vi "Divide Images.vi"(0 "image in":refnum<class "MSC Image.lvclass">, 1 "image 2 in":refnum<class "MSC Image.lvclass">, 2 "Scalar":dbl=1.0, 5 "error in (no error)":errorcluster) -> (14 "image out":refnum<class "MSC Image.lvclass">, 15 "image 2 out":refnum<class "MSC Image.lvclass">, 19 "error out":errorcluster)   [LabVIEW 2016, in "MSC Image.lvclass"]
doc: "image = image / image 2 / Scalar"
uses:
  MSC Image.lvclass
  Dependencies/x86/MSC I Process32.dll
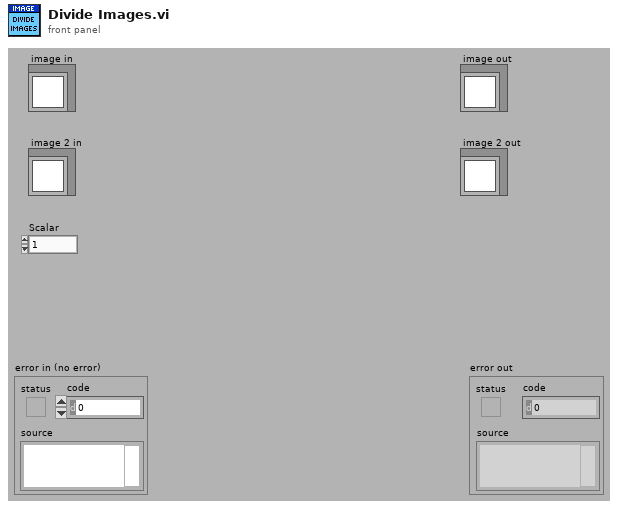
[diagram p1: front panel]
types:
  T1 = typedef "Image.ctl" = cluster{"Pointer":u64, "Size":T2, "Image Type":T3, "Time Stamp":timestamp, "Variant":variant}
  T2 = typedef "Size.ctl" = cluster{"Cols":i32, "Rows":i32}
  T3 = typedef "Image Type.ctl" = i32
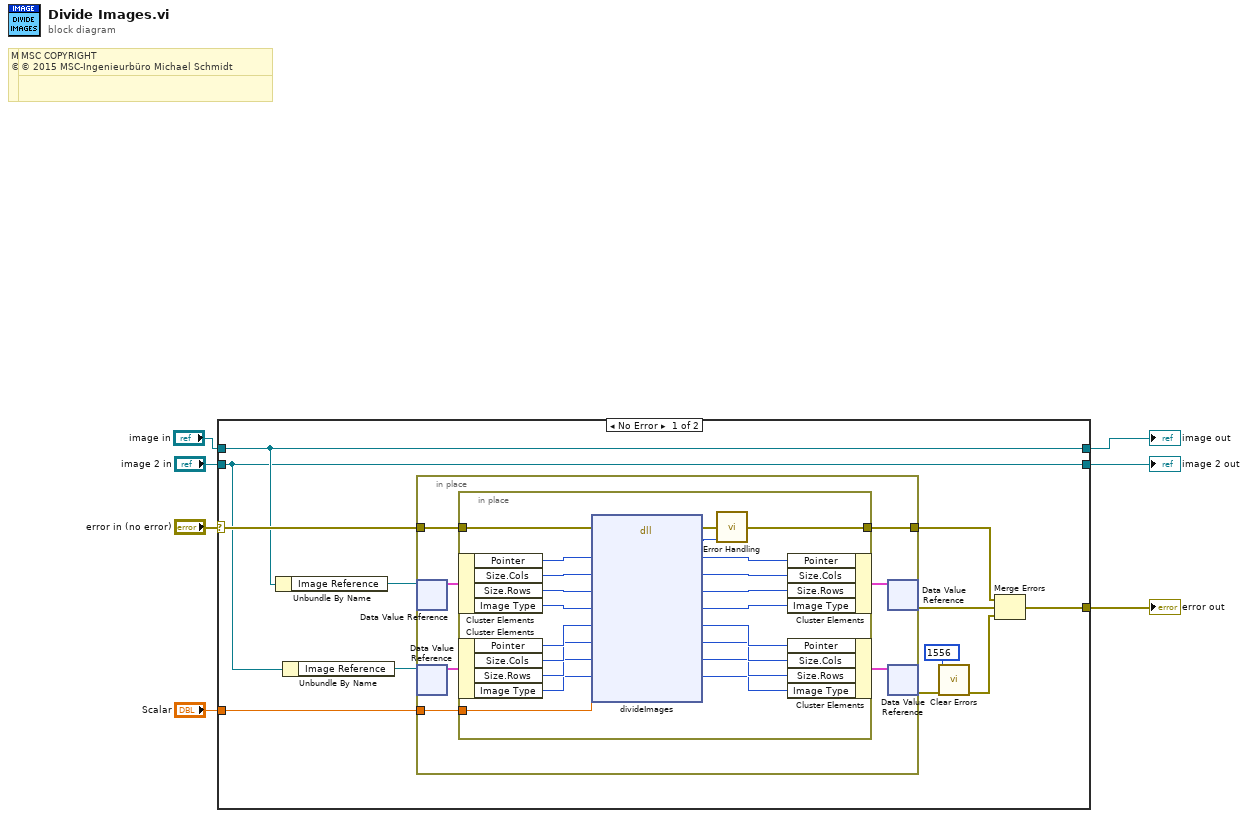
[diagram p0: block diagram]
diagram:
  # "MSC COPYRIGHT\n© 2016 MSC-Ingenieurbüro Michael Schmidt"
  # "MSC COPYRIGHT\n© 2016 MSC-Ingenieurbüro Michael Schmidt"
  # "MSC COPYRIGHT\n© 2015 MSC-Ingenieurbüro Michael Schmidt"
  # "MSC COPYRIGHT\n© 2015 MSC-Ingenieurbüro Michael Schmidt"
  n1 = case shown="No Error" "error in (no error)" {
    selector: "error in (no error)" -> [w16 w50]
    tunnel: [w19 w50] -> w3
    tunnel: [w12 w49] -> w6
    tunnel: "image in" -> [w15 w48]
    tunnel: "image 2 in" -> [w12 w49]
    tunnel: [w15 w48] -> w7
    tunnel: "Scalar" -> [w11 _]
    frame No Error {
      n2 = Unbundle By Name(w15) -> ("Image Reference"=w14:refnum<data-value>)
      n3 = Unbundle By Name(w12) -> ("Image Reference"=w13:refnum<data-value>)
      n4 = in-place {
        in-place-border: w16 -> [w24]
        in-place-border: [w23] -> w18
        in-place-border: w11 -> [w20]
        n5 = in-place-dvr #1(w14) -> (w25:T1)  [unwired: 1 out]
        n6 = in-place-dvr #2(w13) -> (w22:T1)  [unwired: 1 out]
        n7 = in-place {
          in-place-border: w24 -> [w28]
          in-place-border: [w47] -> w23
          in-place-border: w20 -> [w27]
          n8 = in-place-cluster #3(w25) -> ("Pointer"=w46:u64, "Size.Cols"=w45:i32, "Size.Rows"=w44:i32, "Image Type"=w43:T3)
          n9 = in-place-cluster #4(w22) -> ("Pointer"=w42:u64, "Size.Cols"=w41:i32, "Size.Rows"=w40:i32, "Image Type"=w39:T3)
          n10 = dll-call lib="C:/Users/MSC/LabVIEW Projekte/LV 2014/MSC I-Process/user.lib/MSC-I Process/Dependencies/x86/MSC I Process*.dll" fn="divideImages"(error in=w28, "pointer"=w46, "cols"=w45, "rows"=w44, "type"=w43, "pointer2"=w42, "cols2"=w41, "rows2"=w40, "type2"=w39, "scalar"=w27) -> (error out=w29:errorcluster, "error"=w30:i32, "pointer"=w34:u64, "cols"=w33:i32, "rows"=w32:i32, "type"=w31:i32, "pointer2"=w38:u64, "cols2"=w37:i32, "rows2"=w36:i32, "type2"=w35:i32)  [unwired: 3 in, 1 out]
          n11 = call "Error Handling.vi"("error in (no error)"=w29, "return type"=w30) -> ("error out"=w47:errorcluster)  [unwired: 12 in, 1 out]
          n12 = in-place-cluster #3("Pointer"=w34, "Size.Cols"=w33, "Size.Rows"=w32, "Image Type"=w31) -> (w26:T1)
          n13 = in-place-cluster #4("Pointer"=w38, "Size.Cols"=w37, "Size.Rows"=w36, "Image Type"=w35) -> (w21:T1)
        }
        n14 = in-place-dvr #1(w26) -> (w17:errorcluster)  [unwired: 1 out]
        n15 = in-place-dvr #2(w21) -> (w9:errorcluster)  [unwired: 1 out]
      }
      n16 = call <vilib>:"Clear Errors.vi"("error in (no error)"=w9, "specific error code to clear (0: all)"=1556) -> ("error out"=w8:errorcluster)  [unwired: 4 in, 1 out]
      n17 = Merge Errors(w18, w17, w8) -> (w19:errorcluster)
    }
    frame Error {
    }
  }
  "error out" <- w3
  "image out" <- w7
  "image 2 out" <- w6
